vi "题目6.vi"   [LabVIEW 2017]
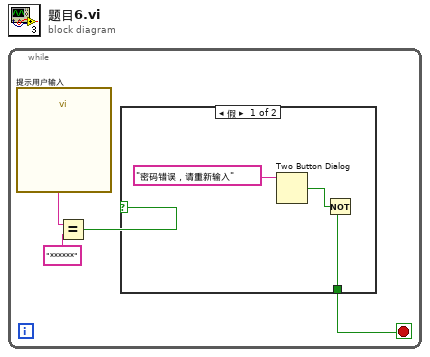
[diagram p0: block diagram]
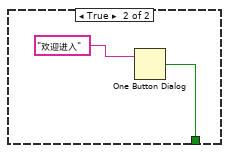
[diagram p2: hidden frame]
diagram:
  n1 = while {
    stop <- w4 stop-if-true
    n2 = call "提示用户输入"() -> ("请输入密码"=w1:string)  [unwired: 17 in, 2 out]
    n3 = Equal?(x=w1, y="******") -> (x = y?=w2:bool)
    n4 = case shown="假" w2 {
      tunnel: [w6 w8] -> w4
      frame False {
        n5 = Two Button Dialog(message="密码错误，请重新输入" ("消息")) -> (T button?=w5:bool)  [unwired: 2 in]
        n6 = Not(x=w5) -> (.not. x?=w6:bool)
      }
      frame True {
        n7 = One Button Dialog(message="欢迎进入" ("消息")) -> (true=w8:bool)  [unwired: 1 in]
      }
    }
  }
